vi "List Subsystems.vi"(8 "error in (no error)":errorcluster) -> (0 "error out":errorcluster, 2 "Subsystems":refnum<class "SMO.lvclass">[](array[class]))   [LabVIEW 2013, in "Registry-SMO.lvclass"]
uses:
  Registry-SMO.lvclass
  SMO/SMO.lvclass
  Registry-SMO.lvclass/Registry-SMO.ctl
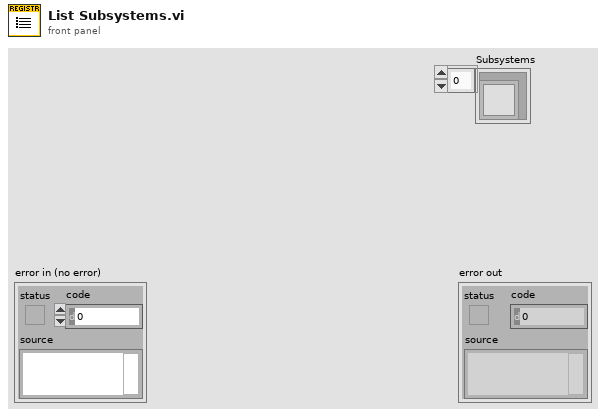
[diagram p1: front panel]
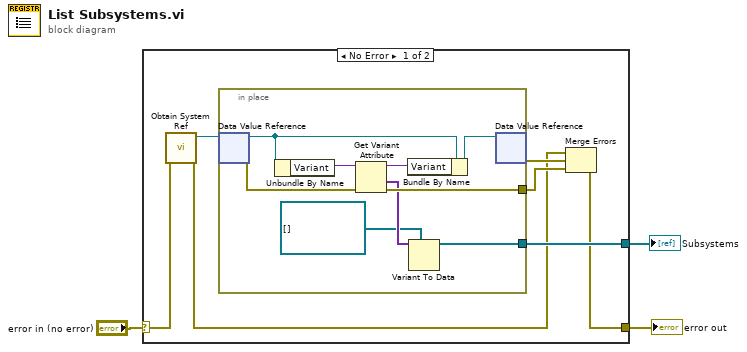
[diagram p0: block diagram]
diagram:
  n1 = case shown="No Error" "error in (no error)" {
    selector: "error in (no error)" -> [w6 w20]
    tunnel: [w4 w20] -> w2
    tunnel: [w8 _] -> w1
    frame No Error {
      n2 = call "Obtain System Ref.vi"("error in (no error)"=w6) -> ("error out"=w5:errorcluster, "JKI SMO System"=w7:refnum<data-value>)  [unwired: 9 in]
      n3 = in-place {
        in-place-border: [w14] -> w9
        in-place-border: [w11] -> w8
        n4 = in-place-dvr #1(w7) -> (w19:refnum<class "Registry-SMO.lvclass">, w15:errorcluster)
        n5 = Unbundle By Name(w19) -> ("Variant"=w17:variant)
        n6 = Get Variant Attribute(Variant=w17, error in=w15) -> (duplicate Variant=w16:variant, values=w13:variant[], error out=w14:errorcluster)  [unwired: 2 in, 1 out]
        n7 = Bundle By Name(cluster=w19, "Variant"=w16) -> (w18:refnum<class "Registry-SMO.lvclass">)
        n8 = Variant To Data(type=refnum<class "SMO.lvclass">[] [], Variant=w13) -> (data=w11:refnum<class "SMO.lvclass">[])  [unwired: 1 in, 1 out]
        n9 = in-place-dvr #1(w18) -> (w10:errorcluster)  [unwired: 1 out]
      }
      n10 = Merge Errors(w5, w10, w9) -> (w4:errorcluster)
    }
    frame Error {
    }
  }
  "error out" <- w2
  "Subsystems" <- w1
